vi "AlliGator Open Single Image.vi"(6 "Interactive?":bool, 8 "Error In":errorcluster, 9 "Image Type":T1, 10 "Image Path in":path, 11 "Image Refnum in":T2) -> (0 "Error Out":errorcluster, 1 "Message":string, 2 "Image Path out":path, 3 "Image Refnum out":T2)   [LabVIEW 2021, in "AlliGator Files.lvlib"]
doc: "Opens a single Mask or White Light image."
uses:
  AlliGator Files.lvlib
  <vilib>/vision/Image Controls.llb/IMAQ Image.ctl
  Source Image/AlliGator Image Type.ctl
  Settings/AlliGator Settings List.ctl
  Source Image/AlliGator Image Binning Options.ctl
  Globals, Variables, Constants/AlliGator Variables List.ctl
  c206d31c-d4ad-4794-9a1a-bb755f8f8898.vi
  Variant/Variant to Data/Variant to Boolean.vi
  <vilib>/Utility/error.llb/Error Cluster From Error Code.vi
  Variant/Variant to Data/Variant to Path.vi
  <vilib>/ErrorRing/Error Ring.xnode
  Source Image/AlliGator Source Image.lvlib
  Settings/AlliGator Settings.lvlib
  Variant/Variant to Data/Variant to Data.lvlib
  <vilib>/vision/NI_Vision_Development_Module.lvlib
  Globals, Variables, Constants/AlliGator Globals, Variables & Constants.lvlib
  Error/Error.lvlib
panel:
  # "see the AlliGator License on the block diagram (Ctrl+E or Window:Show Block Diagram)"
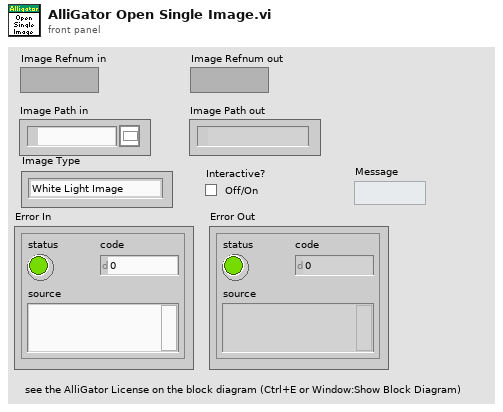
[diagram p1: front panel]
types:
  T1 = typedef "AlliGator Source Image.lvlib/AlliGator Image Type.ctl" = enum16{"White Light Image", "Mask Image"}
  T2 = typedef "IMAQ Image.ctl" = refnum<image>
  T3 = typedef "AlliGator Source Image.lvlib/AlliGator Image Binning Options.ctl" = cluster{"Use Image Binning":bool, "X Bin":i32, "Y Bin":i32}
  T4 = typedef "AlliGator Settings.lvlib/AlliGator Settings List.ctl" = enum16{"GUI:Visible Settings Tab", "GUI:Last Run Version", "Source Image:Use Image Histogram for Contrast", "Source Image:Low Count Pixels Rejection Options", "Source Image:High Count Pixels Rejection Options", "Source Image:Use Image Brightness", "Source Image:Blend Overlay with Image Background", "Source Image:Use Fixed ROI Diameter", "Source Image:ROI Diameter", "Source Image:ROI Center Color", "Source Image:Peak Threshold", "Source Image:Intensity Threshold", "Source Image:Image Binning Options", "Source Image:Image Smoothing Options", "Source Image:Image Histogram Active", "Source Image:Invert Binary Mask", "Source Image:Hot Pixel Removal", "Source Image:Overlay Analyzed ROI Center", "Source Image:Auto-Adjust Contrast", "Source Image:Histogram Lower Percentile", "Source Image:Histogram Upper Percentile", "Source Image:Save Source Image", "Source Image:Scale Bar Options", "Source Image:Image Resolution (Pixel Size)", "Source Image:Flatfield Correction", "Source Image:Show Dead Left Columns Correction", "Source Image:Dead Left Columns Correction", "Source Image:Image Pre-Processing Operations Order", "Source Image:Overlay ROI Median", "Source Image:Median Overlay Color", "Data Information:Gate Width", "Data Information:Nanotime Gate Separation", "Data Information:Macrotime Gate Separation", "Data Information:Gate Step", "Data Information:# Gates", "Data Information:Gate Image Exposure", "Data Information:Gate Image Integration", "Data Information:Gates to Skip", "Data Information:Gates to Keep", "Data Information:Define Gates to", "Data Information:Channel Name", "Data Information:Available Channel Names", "Data Information:Channel Arithmetic", "Data Information:Background File Subtraction", "Data Information:Background File", "Data Information:Background Scaling Factor", "Data Information:Background Pile-up Correction", "Data Information:Background Pixel Well Capacity", "Data Information:Laser Period", "Data Information:SYNC Period", "Data Information:Pile-up Correction", "Data Information:Pixel Well Capacity", "Data Information:Dataset Scaling Factor", "Fluorescence Decay_Decay Pre-Processing:Reverse Gates", "Fluorescence Decay_Decay Pre-Processing:Verbose Decay Pre-Processing", "Fluorescence Decay_Decay Pre-Processing:Use Decay Pre-Processing", "Fluorescence Decay_Decay Pre-Processing:Background Subtraction", "Fluorescence Decay_Decay Pre-Processing:Background Definition Range", "Fluorescence Decay_Decay Pre-Processing:Baseline Subtraction Method", "Fluorescence Decay_Decay Pre-Processing:Decay Pre-Processing Operations Order", "Fluorescence Decay_Decay Pre-Processing:Smoothing Parameter", "Fluorescence Decay_Decay Pre-Processing:Shift Decay", "Fluorescence Decay_Decay Pre-Processing:Decay Shift Parameters", "Fluorescence Decay_Decay Pre-Processing:Fold Decay", "Fluorescence Decay_Decay Pre-Processing:# Folds", "Fluorescence Decay_Decay Pre-Processing:1-Normalize Decay", "Fluorescence Decay_Decay Pre-Processing:[0-1]-Normalize Decay", "Fluorescence Decay_Decay Pre-Processing:Smoothen Decay", "Fluorescence Decay_Decay Pre-Processing:Extrapolate Decay", "Fluorescence Decay_Decay Pre-Processing:Use Periodicity", "Fluorescence Decay_Decay Pre-Processing:Use Cursors", "Fluorescence Decay_Decay Pre-Processing:Tail Fraction", "Fluorescence Decay_Decay Pre-Processing:Head Fraction", "Fluorescence Decay_Decay Pre-Processing:Additional Points", "Fluorescence Decay_Decay Pre-Processing:Straighten Decay", "Fluorescence Decay_Decay Pre-Processing:Constant Background", "Fluorescence Decay_Decay Pre-Processing:Pixel-Normalize Decay", "Fluorescence Decay_Advanced Analysis:Extract IRF instead of Decay", "Fluorescence Decay_Advanced Analysis:IRF Extraction Options", "Fluorescence Decay_Advanced Analysis:IRF Optimization Options", "Fluorescence Decay_Advanced Analysis:Square Pulse Options", "Fluorescence Decay_Advanced Analysis:IRF Order", "Fluorescence Decay_Advanced Analysis:IRF Time Constants", "Fluorescence Decay_Advanced Analysis:Wavelet Analysis Options", "Fluorescence Decay_Advanced Analysis:Average Lifetime Options", "Fluorescence Decay_Fit Options:Fit Options", "Fluorescence Decay_Fit Options:Use Legacy Fitting Approach", "Fluorescence Decay_Fit Options:Use Data Information Laser Period", "Fluorescence Decay_Fit Parameters:Displayed Fit Parameters", "Fluorescence Decay_Fit Parameters:Fit Parameter Constraints", "Fluorescence Decay_Fit Parameters:Export Tabulated Results", "Fluorescence Decay_Fit Parameters:MLE Baseline Offset Type", "Fluorescence Decay_Fit Parameters:MLE Baseline Offset", "Fluorescence Decay_Fit Parameters:Guess Parameter Names", "Fluorescence Decay_Fit Parameters:Guess Parameter Values", "Fluorescence Decay_Fit Parameters:Guess Parameters Options", "Fluorescence Decay_Styles:Show Last Decay Only", "Fluorescence Decay_Styles:Decay Graph Color Array", "Fluorescence Decay:Decay Graph Active", "Fluorescence Decay Statistics:Min Peak Value", "Fluorescence Decay Statistics:Reject Low Decay Peak Pixels", "Fluorescence Decay Statistics:Reject High Decay Peak Pixels", "Fluorescence Decay Statistics:Max Peak Value", "Time Traces:Use File Timestamp", "Time Traces:Time Step", "Time Traces:Use Intensity Correction File", "Time Traces:Intensity Correction File", "Phasor Plot:Phasor Plot Smoothing Options", "Phasor Plot:Phasor Plot Size", "Phasor Plot:Phasor Plot Graphics Options", "Phasor Plot:Cumulative Phasor Plot", "Phasor Plot:Use Phasor Brightness", "Phasor Plot:Blend Overlay with Phasor Background", "Phasor Plot:Save Phasor Plot", "Phasor Plot:Show References", "Phasor Plot:Phasor Ratio Decay Range", "Phasor Plot:Exponential Fading", "Phasor Plot:Phasor Ratio Reference Colors", "Phasor Plot:Reference Radius", "Phasor Plot:Show Color Map Vertices", "Phasor Plot:Phasor Plot Active", "Phasor Plot:Phasor Ratio Color Map Type", "Phasor Plot:Phasor Ratio Color Map", "Phasor Plot:Phasor Ratio Display Range", "Phasor Plot:Selected Image ROI(s)", "Phasor Plot:All Image ROIs", "Phasor Plot:Selected Phasor Plot ROI(s)", "Phasor Plot:All Phasor Plot ROIs", "Phasor Plot:Phasor Ratio Color-Coded Quantity", "Phasor Plot:Store Phasor Harmonics", "Phasor Plot:Draw Reference Segment", "Phasor Plot:User-Defined Quantity", "Phasor Graph:Phasor Frequency", "Phasor Graph:Phasor Ratio Type", "Phasor Graph:Pixel-level Phasor Computation", "Phasor Graph:Save Phasor Graph", "Phasor Graph:Phasor Graph Active", "Phasor Graph:Phasor SDV Options", "Phasor Calibration:Use Backup Calibration if needed", "Phasor Graph:Define Shortest Lifetime as", "Phasor Calibration:Backup Calibration Type", "Phasor Calibration:Calibration Type", "Phasor Calibration:Calibration Lifetime", "Phasor Calibration:Calibration Map Algorithm", "Single-Exponential Phasor Locus (SEPL):Gate Parameters", "Single-Exponential Phasor Locus (SEPL):User-defined Gate", "Single-Exponential Phasor Locus (SEPL):User-defined IRF", "Single-Exponential Phasor Locus (SEPL):Phasor Parameters", "Single-Exponential Phasor Locus (SEPL):Decay & IRF Parameters", "Single-Exponential Phasor Locus (SEPL):Display Parameters", "Lifetime Analysis:Decay Analysis Parameters", "Lifetime Analysis:Lifetime Map Active", "Plugins:Python Settings", "Miscellaneous:Verbose Mode", "Miscellaneous:Beep after Script", "Miscellaneous:Saved Image File Format", "Miscellaneous:Exported Gate Image Settings", "Miscellaneous:Include Loading in Timing", "Miscellaneous:Verbose Settings Mode", "Miscellaneous:Histogram Options", "Miscellaneous:Beep on Error", "Miscellaneous:# Logical Processors Used", "Miscellaneous:ROI Description Max Characters", "Miscellaneous:Verbose Error Mode", "Miscellaneous:Transparent Mask Color"}
  T5 = typedef "AlliGator Globals, Variables & Constants.lvlib/AlliGator Variables List.ctl" = enum16{"---- GUI ----", "GUI:Initialization Status", "GUI:State Indicators Refnum", "GUI:Original AlliGator Menu Items", "GUI:Current Action Loop State", "GUI:Script in progress", "GUI:Playback", "GUI:Loop Playback", "GUI:Search ROI Used", "GUI:Search ROI", "Decay Graph Max Legend Size", "Intensity Graph Max Legend Size", "Decay Statistics Graph Max Legend Size", "Phasor Graph Max Legend Size", "Phasor Ratio Graph Max Legend Size", "Lifetime Graph Max Legend Size", "---- Files ----", "Files:Export Dataset Frames as Individual Files", "Files:Show Batch Export Help Balloons", "Files:Frames in Dataset", "Files:ptu File Frame Start Indices", "Files:Current Frame in Dataset", "Files:Current Frame Timestamp", "Files:Dataset Loaded", "Files:Dataset Metadata", "Files:Dataset Channel", "Files:Dataset Data Description", "Files:Background Dataset Metadata", "Files:Background Dataset Channel", "Files:Background Dataset Data Description", "Files:Background File Subtraction", "Files:Background File Path", "Files:Background File Pile-up Correction", "Files:Background File Pixel Well Capacity", "Files:Background File Scaling Factor", "Files:Current Dataset Load Settings", "Files:Dataset Path", "Files:ICCD-specific Information", "Files:Macrotime Gate Separation", "------ Python Plugins ------", "Python Plugins:Information", "Python Plugins:Python Session", "Python Plugins:Valid Python Session?", "---- Source Image ----", "Source Image:ROIs", "Source Image:Current ROI", "Source Image:ROI Event Refnum", "X_Source Image Display Range", "X_Source Image Palette Information", "X_Type of Displayed Image", "X_Time Gate Slider", "Source Image:Palette List", "Source Image:Scale", "Source Image:ROI Overlay Color", "Source Image:Overlay to Erase", "Source Image:Is Displayed Image Accumulated", "Source Image:White Light Image Modified", "Source Image:Mask Image Modified", "---- Image Profile Window ----", "Image Profile:Window Event Refnum", "Image Profile:IntensityType", "Image Profile:Intensity Average Type", "Image Profile:Intensity-weighted SDV", "Image Profile:Box Profile Type", "Image Profile:Window Open", "Image Profile:Plotted Fit Parameter", "------ Phasor Graph -------", "Phasor Graph:Show Line", "---- Phasor Plot ---", "Phasor Plot:Parameters Changed", "Phasor Plot:FLI Dataset Modified since last Calculation", "Phasor Harmonics Data", "Selected Phasor Harmonics", "Phasor Harmonic Manager Event Refnum", "Phasor Plot:ROIs", "Phasor Plot:Current ROI", "Phasor Plot:ROI Event Refnum", "Phasor Plot:Image Reference Points", "Phasor Plot:Computed", "Phasor Plot:Palette Information", "Phasor Plot:Palette List", "Phasor Plot:Phasor Ratio Palette Information", "Phasor Plot:Phasor Ratio Palette List", "Phasor Plot:Image Scale", "Phasor Plot:Image Overlay to Erase", "Phasor Plot:Image Elements to Update", "Phasor Plot:Current Calculation Parameters", "Phasor Plot:Current Calibration Options", "Phasor Plot:Reset Cumulated Phasor Plot", "Phasor Plot:Reference 1", "Phasor Plot:Lifetime Reference 1", "Phasor Plot:Reference 1 Frequency", "Phasor Plot:Reference 2", "Phasor Plot:Lifetime Reference 2", "Phasor Plot:Reference 2 Frequency", "---- Decay Analysis ----", "Number of Selected Decays to Fit", "LS Fit Results", "LAR Fit Results", "BS Fit Results", "Last Decay Max - Min", "Best Fit Parameters", "Best Fit Parameter Names", "Actual Size X", "Actual Size Y", "Binning X", "Binning Y", "Actual # Gates", "Dataset Number", "Gates to...", "Gates Skipped", "Gates to keep", "Gate Step", "Gate Separation", "Reversed Gates", "Pile-up Correction", "Pixel Well Capacity", "Background Subtracted", "Background Subtraction Method", "Background Definition Range", "Background File (deprecated)", "Number of Dataset Accumulated", "Array of Accumulated Dataset Paths", "Do Averaged Datasets", "Destination File Path", "Process Plot Target", "Use 1/D as Phasor Frequency", "---- Decay Fit Parameter Map -----", "Decay Fit Parameter Map:Palette Information", "Decay Fit Parameter Map:Palette List", "---- Parameter Map ----", "Parameter Map:Palette Information", "Parameter Map:Palette List", "------- Local Decay Window ---------", "Local Decay Graph Window:Event Refnum", "Local Decay Graph Window:Use normalized IRF for convolution", "----- Miscellaneous ----", "Misc:Skippable Dialog Windows Status"}
  T6 = typedef "Image Type" = u32
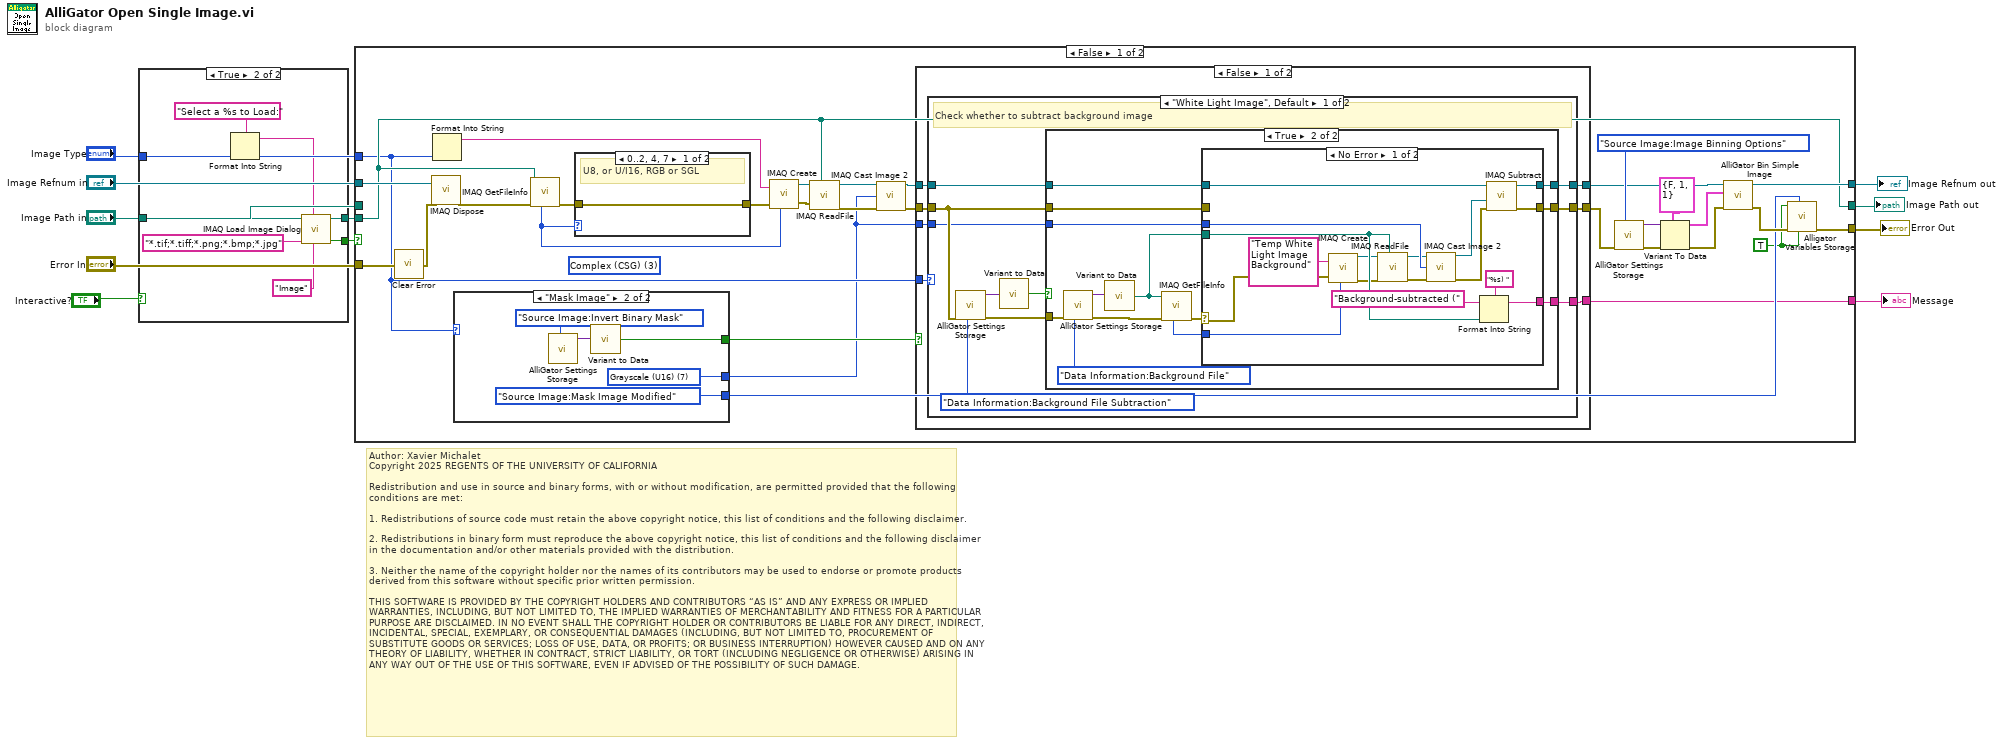
[diagram p0: block diagram]
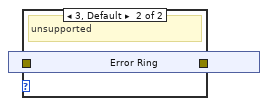
[diagram p3: hidden frame]
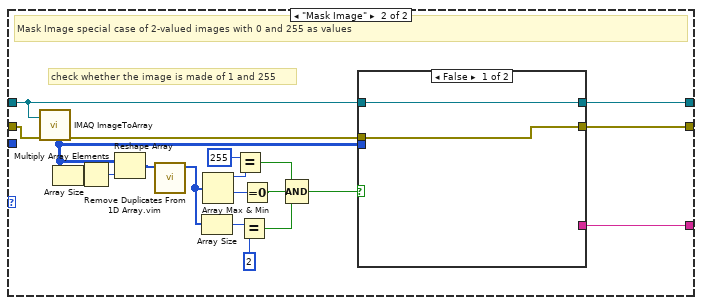
[diagram p6: hidden frame]
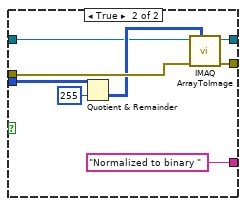
[diagram p7: hidden frame]
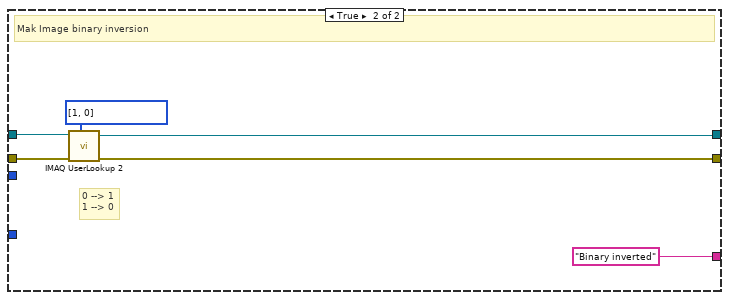
[diagram p8: hidden frame]
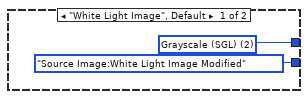
[diagram p9: hidden frame]
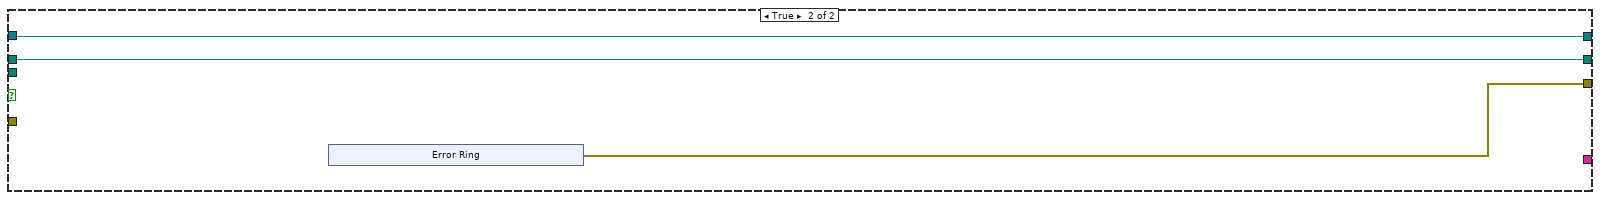
[diagram p10: hidden frame]
diagram:
  # "Author: Xavier Michalet\nCopyright 2025 REGENTS OF THE UNIVERSITY OF CALIFORNIA\n\nRedistribution and use in source and binary forms, with or without modification, are permitted provided that the following conditions are met:\n\n1. Redistributions of source code must retain the above copyright notice, this list of conditions and the following disclaimer.\n\n2. Redistributions in binary form must reproduce the above copyright notice, this list of conditions and the following disclaimer in the documentation and/or other materials provided with the distribution.\n\n3. Neither the name of the copyright holder nor the names of its contributors may be used to endorse or promote products derived from this software without specific prior written permission.\n\nTHIS SOFTWARE IS PROVIDED BY THE COPYRIGHT HOLDERS AND CONTRIBUTORS “AS IS” AND ANY EXPRESS OR IMPLIED WARRANTIES, INCLUDING, BUT NOT LIMITED TO, THE IMPLIED WARRANTIES OF MERCHANTABILITY AND FITNESS FOR A PARTICULAR PURPOSE ARE DISCLAIMED. IN NO EVENT SHALL THE COPYRIGHT HOLDER OR CONTRIBUTORS BE LIABLE FOR ANY DIRECT, INDIRECT, INCIDENTAL, SPECIAL, EXEMPLARY, OR CONSEQUENTIAL DAMAGES (INCLUDING, BUT NOT LIMITED TO, PROCUREMENT OF SUBSTITUTE GOODS OR SERVICES; LOSS OF USE, DATA, OR PROFITS; OR BUSINESS INTERRUPTION) HOWEVER CAUSED AND ON ANY THEORY OF LIABILITY, WHETHER IN CONTRACT, STRICT LIABILITY, OR TORT (INCLUDING NEGLIGENCE OR OTHERWISE) ARISING IN ANY WAY OUT OF THE USE OF THIS SOFTWARE, EVEN IF ADVISED OF THE POSSIBILITY OF SUCH DAMAGE."
  n1 = case shown="True" "Interactive?" {
    tunnel: [_ w20] -> w11
    tunnel: "Image Path in" -> [w12 w19]
    tunnel: [w12 w18] -> w6
    tunnel: "Image Type" -> [_ w15]
    frame False {
    }
    frame True {
      n2 = Format Into String(format string="Select a %s to Load:" ("Prompt"), w15) -> (resulting string=w17:string)  [unwired: 2 in, 1 out]
      n3 = call "IMAQ Load Image Dialog"("Pattern Label"="Image", "Prompt"=w17, "Pattern"="*.tif;*.tiff;*.png;*.bmp;*.jpg", "Start Path"=w19) -> ("Cancelled?"=w20:bool, "Path"=w18:path)  [unwired: 5 in, 1 out]
    }
  }
  n4 = case shown="False" w11 {
    tunnel: "Image Refnum in" -> [w52 w155]
    tunnel: [w49 w155] -> w9
    tunnel: "Image Path in" -> [_ w154]
    tunnel: [w31 w154] -> w7
    tunnel: w6 -> [w31 _]
    tunnel: "Error In" -> [w30 _]
    tunnel: [w38 w153] -> w4
    tunnel: "Image Type" -> [w25 _]
    tunnel: [w23 _] -> w1
    frame False {
      (unwired) T6 3 items=["Grayscale (U8)", "Grayscale (I16)", "Grayscale (SGL)", "Complex (CSG)", "RGB (U32)", "HSL (U32)", "RGB (U64)", "Grayscale (U16)"] ("Image Type")
      w36 = TRUE ("Get(F)/Set")
      n5 = call "Clear Error.vi"("Error In"=w30) -> ("no Error Out"=w21:errorcluster)  [unwired: 8 in]
      n6 = call "IMAQ Dispose"("Image"=w52, "error in (no error)"=w21) -> ("error out"=w26:errorcluster)  [unwired: 4 in]
      n7 = Format Into String(w25) -> (resulting string=w29:string)  [unwired: 3 in, 1 out]
      n8 = case shown="\"Mask Image\"" w25 {
        tunnel: [_ w150] -> w42
        tunnel: [AlliGator_Variables_List."Source Image:White Light Image Modified" ("Alligator Variable") AlliGator_Variables_List."Source Image:Mask Image Modified" ("Alligator Variable")] -> w37
        tunnel: [w146 w148] -> w22
        frame "White Light Image", Default {
          w146 = T6 2 items=["Grayscale (U8)", "Grayscale (I16)", "Grayscale (SGL)", "Complex (CSG)", "RGB (U32)", "HSL (U32)", "RGB (U64)", "Grayscale (U16)"] ("Image Type")
        }
        frame "Mask Image" {
          w148 = T6 7 items=["Grayscale (U8)", "Grayscale (I16)", "Grayscale (SGL)", "Complex (CSG)", "RGB (U32)", "HSL (U32)", "RGB (U64)", "Grayscale (U16)"] ("Image Type")
          n9 = call "AlliGator Settings Storage.vi"("AlliGator Settings List"=AlliGator_Settings_List."Source Image:Invert Binary Mask") -> ("Variant Data out"=w152:variant)  [unwired: 9 in, 1 out]
          n10 = call-poly "Variant to Data.vi"("Variant"=w152) -> ("Value"=w150:bool)  [unwired: 8 in]
        }
      }
      n11 = call "IMAQ GetFileInfo"("error in (no error)"=w26, "File Path"=w31) -> ("error out"=w28:errorcluster, "Image Type"=w24:T6)  [unwired: 3 in, 5 out]
      n12 = case shown="0..2, 4, 7" w24 {
        tunnel: w28 -> [w53 _]
        tunnel: [w53 w54] -> w27
        frame 0..2, 4, 7 {
          # "U8, or U/I16, RGB or SGL"
        }
        frame 3, Default {
          # "unsupported"
          n13 = xnode "Error Ring"() -> ("error out"=w54:errorcluster)
        }
      }
      n14 = call "IMAQ Create"("Image Name"=w29, "Image Type"=w24, "error in (no error)"=w27) -> ("New Image"=w51:T2, "error out"=w50:errorcluster)  [unwired: 2 in]
      n15 = call "IMAQ ReadFile"("File Path"=w31, "error in (no error)"=w50, "Image"=w51) -> ("error out"=w35:errorcluster, "Image Out"=w34:T2)  [unwired: 4 in, 3 out]
      n16 = call "IMAQ Cast Image 2"("Image Src"=w34, "Image Type"=w22, "error in (no error)"=w35) -> ("Image Dst Out"=w33:T2, "error out"=w32:errorcluster)  [unwired: 11 in]
      n17 = case shown="False" w42 {
        tunnel: w32 -> [w65 w142]
        tunnel: w33 -> [w64 w144]
        tunnel: [w63 w143] -> w41
        tunnel: [w62 w141] -> w40
        tunnel: w25 -> [w61 _]
        tunnel: [w60 "Binary inverted" ("Message")] -> w23
        tunnel: w22 -> [w59 _]
        frame False {
          n18 = case shown="\"White Light Image\", Default" w61 {
            tunnel: w65 -> [w68 w129]
            tunnel: w64 -> [w72 w116]
            tunnel: [w71 w115] -> w63
            tunnel: [w70 w113] -> w62
            tunnel: [w67 w110] -> w60
            tunnel: w59 -> [w66 _]
            frame "White Light Image", Default {
              # "Check whether to subtract background image"
              n19 = call "AlliGator Settings Storage.vi"("AlliGator Settings List"=AlliGator_Settings_List."Data Information:Background File Subtraction", "Error In"=w68) -> ("Error Out"=w69:errorcluster, "Variant Data out"=w74:variant)  [unwired: 8 in]
              n20 = call-poly "Variant to Data.vi"("Variant"=w74) -> ("Value"=w73:bool)  [unwired: 8 in]
              n21 = case shown="True" w73 {
                tunnel: w72 -> [w77 w84]
                tunnel: [w77 w83] -> w71
                tunnel: [w76 w81] -> w70
                tunnel: w69 -> [w76 w90]
                tunnel: w68 -> [_ w82]
                tunnel: [_ w79] -> w67
                tunnel: w66 -> [_ w78]
                frame False {
                }
                frame True {
                  n22 = call "AlliGator Settings Storage.vi"("AlliGator Settings List"=AlliGator_Settings_List."Data Information:Background File", "Error In"=w90) -> ("Error Out"=w87:errorcluster, "Variant Data out"=w88:variant)  [unwired: 8 in]
                  n23 = call-poly "Variant to Data.vi"("Variant"=w88) -> ("Path"=w80:path)  [unwired: 8 in]
                  n24 = call "IMAQ GetFileInfo"("error in (no error)"=w87, "File Path"=w80) -> ("error out"=w86:errorcluster, "Image Type"=w85:T6)  [unwired: 3 in, 5 out]
                  n25 = case shown="No Error" w86 {
                    selector: w86 -> [w92 _]
                    tunnel: w85 -> [w107 _]
                    tunnel: w84 -> [w106 w109]
                    tunnel: [w104 w109] -> w83
                    tunnel: w82 -> [_ w108]
                    tunnel: [w103 w108] -> w81
                    tunnel: w80 -> [w105 _]
                    tunnel: [w102 _] -> w79
                    tunnel: w78 -> [w101 _]
                    frame No Error {
                      n26 = call "IMAQ Create"("Image Name"="Temp White Light Image Background", "Image Type"=w107, "error in (no error)"=w92) -> ("New Image"=w98:T2, "error out"=w99:errorcluster)  [unwired: 2 in]
                      n27 = call "IMAQ ReadFile"("File Path"=w105, "error in (no error)"=w99, "Image"=w98) -> ("error out"=w96:errorcluster, "Image Out"=w97:T2)  [unwired: 4 in, 3 out]
                      n28 = call "IMAQ Cast Image 2"("Image Src"=w97, "Image Type"=w101, "error in (no error)"=w96) -> ("Image Dst Out"=w95:T2, "error out"=w94:errorcluster)  [unwired: 11 in]
                      n29 = Format Into String(format string="%s) ", initial string="Background-subtracted (" ("Message"), w105) -> (resulting string=w102:string)  [unwired: 1 in, 1 out]
                      n30 = call "IMAQ Subtract"("Image Src A"=w106, "Image Src B"=w95, "error in (no error)"=w94) -> ("Image Dst Out"=w104:T2, "error out"=w103:errorcluster)  [unwired: 4 in]
                    }
                    frame Error {
                    }
                  }
                }
              }
            }
            frame "Mask Image" {
              # "check whether the image is made of 1 and 255"
              # "Mask Image special case of 2-valued images with 0 and 255 as values"
              n31 = call "IMAQ ImageToArray"("error in (no error)"=w129, "Image"=w116) -> ("Image Pixels (U16)"=w112:u16[][], "error out"=w114:errorcluster)  [unwired: 2 in, 3 out]
              n32 = Array Size(array=w112) -> (size(s)=w128:i32[])
              n33 = Multiply Array Elements(1:w128) -> (0:w127:i32)
              n34 = Reshape Array(w112, w127) -> (w126:u16[])
              n35 = call "Remove Duplicates From 1D Array.vim"("array"=w126) -> ("array with duplicates removed"=w123:u16[])  [unwired: 10 in]
              n36 = Array Size(array=w123) -> (size(s)=w125:i32)
              n37 = Array Max & Min(array=w123) -> (max value=w122:u16, min value=w111:u16)  [unwired: 2 out]
              n38 = Equal?(x=u16 255, y=w122) -> (x = y?=w120:bool)
              n39 = Equal?(x=w125, y=2) -> (x = y?=w118:bool)
              n40 = Equal To 0?(x=w111) -> (x = 0?=w119:bool)
              n41 = Compound Arithmetic op=AND(w120, w119, w118) -> (w117:bool)
              n42 = case shown="False" w117 {
                tunnel: w116 -> [w131 w136]
                tunnel: [w131 w135] -> w115
                tunnel: w114 -> [w130 w138]
                tunnel: [w130 w134] -> w113
                tunnel: w112 -> [_ w133]
                tunnel: [_ "Normalized to binary " ("Message")] -> w110
                frame False {
                }
                frame True {
                  n43 = Quotient & Remainder(x=w133, y=u16 255) -> (floor(x/y)=w137:u16[][])  [unwired: 1 out]
                  n44 = call "IMAQ ArrayToImage"("Image Pixels (U16)"=w137, "error in (no error)"=w138, "Image"=w136) -> ("error out"=w134:errorcluster, "Image Out"=w135:T2)  [unwired: 7 in]
                }
              }
            }
          }
        }
        frame True {
          # "0 --> 1\n1 --> 0"
          # "Mak Image binary inversion"
          n45 = call "IMAQ UserLookup 2"("Image Src"=w144, "Lookup Table"=i32[] [1, 0], "error in (no error)"=w142) -> ("Image Dst Out"=w143:T2, "error out"=w141:errorcluster)  [unwired: 4 in]
        }
      }
      n46 = call "AlliGator Settings Storage.vi"("AlliGator Settings List"=AlliGator_Settings_List."Source Image:Image Binning Options", "Error In"=w40) -> ("Error Out"=w47:errorcluster, "Variant Data out"=w48:variant)  [unwired: 8 in]
      n47 = Variant To Data(error in=w47, type=T3 {"Use Image Binning"=FALSE, "X Bin"=1, "Y Bin"=1} ("Image Binning Options"), Variant=w48) -> (data=w44:T3, error out=w45:errorcluster)
      n48 = call "AlliGator Bin Simple Image.vi"("error in (no error)"=w45, "Image Binning Options"=w44, "Refnum in"=w41) -> ("error out"=w39:errorcluster, "Refnum out"=w49:T2)  [unwired: 7 in]
      n49 = call "Alligator Variables Storage.vi"("Get(F)/Set"=w36, "AlliGator Variable"=w37, "Error In"=w39, "Data in"=w36) -> ("Error Out"=w38:errorcluster)  [unwired: 5 in, 2 out]
    }
    frame True {
      n50 = xnode "Error Ring"() -> ("error out"=w153:errorcluster)
    }
  }
  "Image Path out" <- w7
  "Image Refnum out" <- w9
  "Error Out" <- w4
  "Message" <- w1
